vi "PV Change Name.vi"(1 "Input":string) -> (0 "Output":string)   [LabVIEW 2024, in "Pfeiffer Vacuum.lvlib"]
uses:
  <instrlib>/Pfeiffer Vacuum/Pfeiffer Vacuum.lvlib
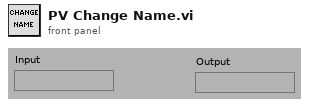
[diagram p1: front panel]
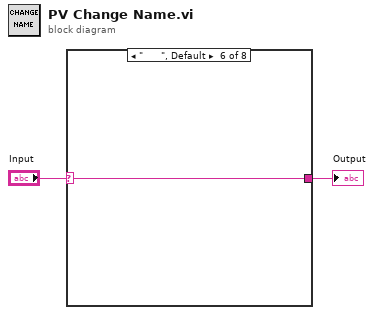
[diagram p0: block diagram]
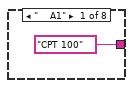
[diagram p2: hidden frame]
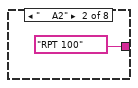
[diagram p3: hidden frame]
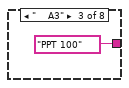
[diagram p4: hidden frame]
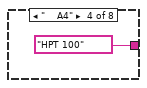
[diagram p5: hidden frame]
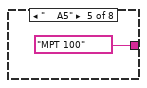
[diagram p6: hidden frame]
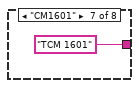
[diagram p7: hidden frame]
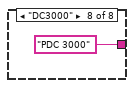
[diagram p8: hidden frame]
diagram:
  n1 = case shown="\"      \", Default" "Input" {
    selector: "Input" -> [_ _ _ _ _ w8 _ _]
    tunnel: ["CPT 100" "RPT 100" "PPT 100" "HPT 100" "MPT 100" w8 "TCM 1601" "PDC 3000"] -> w1
    frame "    A1" {
    }
    frame "    A2" {
    }
    frame "    A3" {
    }
    frame "    A4" {
    }
    frame "    A5" {
    }
    frame "      ", Default {
    }
    frame "CM1601" {
    }
    frame "DC3000" {
    }
  }
  "Output" <- w1
